vi "setPLL_Settings.vi"(0 "Interface in":T3, 5 "PLLgains":T2 {"proportional gain" step=0.125}, 7 "PLLrange":T1={"output high (Inf)"=inf, "output low (-Inf)"=-inf}, 11 "error in":errorcluster) -> (4 "Interface out":T3, 15 "error out":errorcluster)   [LabVIEW 2017, in "ThreePhasePLLInterface.lvlib"]
uses:
  ThreePhasePLLInterface.lvlib
  InterfaceRef.ctl
  <instrlib>/_niInstr/Instruction Framework/v1/Host/Instruction Target/niInstr Instruction Target v1 Host.lvclass
  <instrlib>/_niInstr/Instruction Framework/v1/Host/Instruction Framework Context/niInstr Instruction Framework Context v1 Host.lvclass
  <vilib>/rvi/Analysis/control/PID/Typedef/niFpgaPID_PIGains.ctl
  <vilib>/rvi/Analysis/control/PID/Typedef/niFpgaPID_OutputRange.ctl
  <vilib>/NI/JSON Support for LabVIEW/JSON Data Classes/JSON Helper/To File (Path).vi
  <vilib>/NI/JSON Support for LabVIEW/JSON Data Classes/JSON Helper/JSON Helper.lvclass
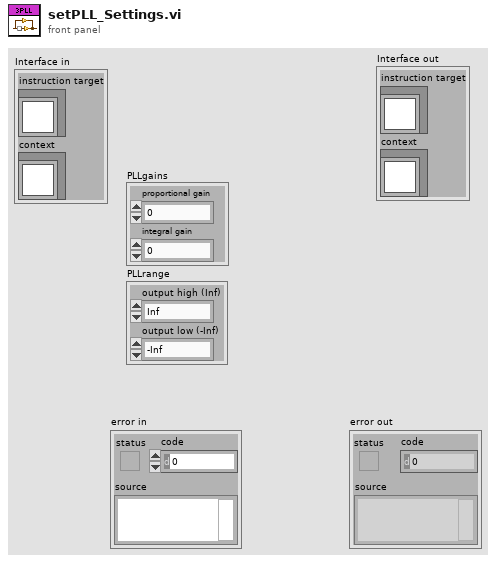
[diagram p1: front panel]
types:
  T1 = typedef "niFpgaPID_OutputRange.ctl" = cluster{"output high (Inf)":sgl, "output low (-Inf)":sgl}
  T2 = typedef "niFpgaPID_PIGains.ctl" = cluster{"proportional gain":sgl, "integral gain":sgl}
  T3 = typedef "ThreePhasePLLInterface.lvlib/InterfaceRef.ctl" = cluster{"instruction target":refnum<class "niInstr Instruction Target v1 Host.lvclass">, "context":refnum<class "niInstr Instruction Framework Context v1 Host.lvclass">}
  T4 = enum16{"open", "replace", "create", "open or create", "replace or create", "replace or create with confirmation"}
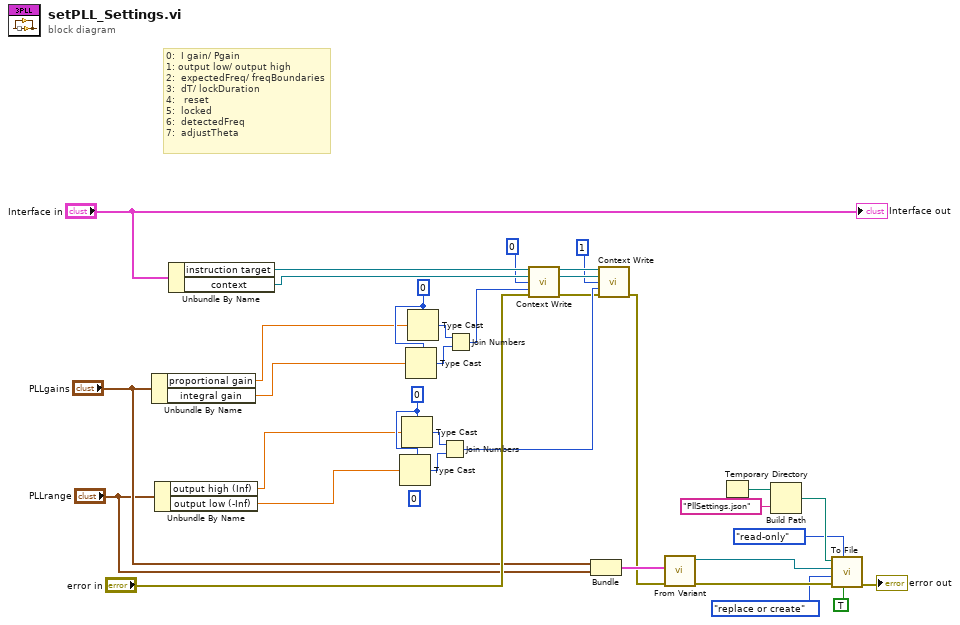
[diagram p0: block diagram]
diagram:
  (unwired) u32 0
  w21 = u32 0
  w30 = u32 0
  # "0:  I gain/ Pgain\n1: output low/ output high\n2:  expectedFreq/ freqBoundaries\n3:  dT/ lockDuration\n4:   reset\n5:  locked\n6:  detectedFreq\n7:  adjustTheta"
  n1 = Unbundle By Name("PLLgains") -> ("proportional gain"=w17:sgl, "integral gain"=w16:sgl)
  n2 = Unbundle By Name("PLLrange") -> ("output high (Inf)"=w15:sgl, "output low (-Inf)"=w14:sgl)
  n3 = Unbundle By Name("Interface in") -> ("instruction target"=w34:refnum<class "niInstr Instruction Target v1 Host.lvclass">, "context"=w33:refnum<class "niInstr Instruction Framework Context v1 Host.lvclass">)
  n4 = Type Cast(type=w21, x=w14) -> (*(type *) &x=w23:u32)
  n5 = Type Cast(type=w21, x=w15) -> (*(type *) &x=w22:u32)
  n6 = Type Cast(type=w30, x=w16) -> (*(type *) &x=w28:u32)
  n7 = Type Cast(type=w30, x=w17) -> (*(type *) &x=w29:u32)
  n8 = Join Numbers(hi=w22, lo=w23) -> ((hi.lo)=w20:u64)
  n9 = Join Numbers(hi=w29, lo=w28) -> ((hi.lo)=w27:u64)
  n10 = call <instrlib>:"Context Write.vi"("instruction target in"=w34, "context in"=w33, "address"=u64 0, "data"=w27, "error in"="error in") -> ("instruction target out"=w25:refnum<class "niInstr Instruction Target v1 Host.lvclass">, "context out"=w24:refnum<class "niInstr Instruction Framework Context v1 Host.lvclass">, "error out"=w18:errorcluster)  [unwired: 8 in]
  n11 = Bundle("PLLgains"="PLLgains", "PLLrange"="PLLrange") -> (w11:cluster{"PLLgains":T2, "PLLrange":T1})  [unwired: 1 in]
  n12 = call <instrlib>:"Context Write.vi"("instruction target in"=w25, "context in"=w24, "address"=u64 1, "data"=w20, "error in"=w18) -> ("error out"=w10:errorcluster)  [unwired: 8 in, 2 out]
  n13 = call <vilib>:"From Variant.vi"("error in (no error)"=w10, "Variant"=w11) -> ("error out"=w8:errorcluster, "JSON out"=w9:refnum<class "JSON Null.lvclass">)  [unwired: 8 in]
  n14 = Temporary Directory() -> (w6:path)
  n15 = Build Path(base path=w6, name or relative path="PllSettings.json") -> (appended path=w4:path)
  n16 = call-poly <vilib>:"To File.vi"("Pretty Print?"=TRUE, "access (0:read/write)"=enum16{"read/write", "read-only", "write-only"}."read-only", "error in (no error)"=w8, "operation (0:open)"=T4."replace or create", "JSON Datatype in"=w9, "file path"=w4) -> ("error out"=→"error out":errorcluster)  [unwired: 5 in]
  "Interface out" <- "Interface in"
